vi "CreateTableDB.vi"(8 "error in (no error)":errorcluster) -> (0 "error out":errorcluster)   [LabVIEW 2020, in "Settings.lvlib"]
uses:
  Settings.lvlib
  <vilib>/drjdpowell/SQLite Library/SQL Connection/Open (path).vi
  <vilib>/drjdpowell/SQLite Library/SQL Connection/Open (string).vi
  <vilib>/AdvancedString/Path To Command Line String.vi
  <vilib>/drjdpowell/SQLite Library/SQL Connection/Execute SQL (No results).vi
  <vilib>/drjdpowell/SQLite Library/SQL Connection/Connection.lvclass
  <vilib>/drjdpowell/SQLite Library/SQLite.lvlib
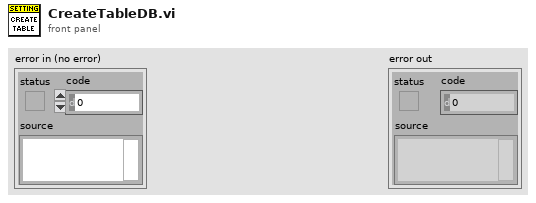
[diagram p1: front panel]
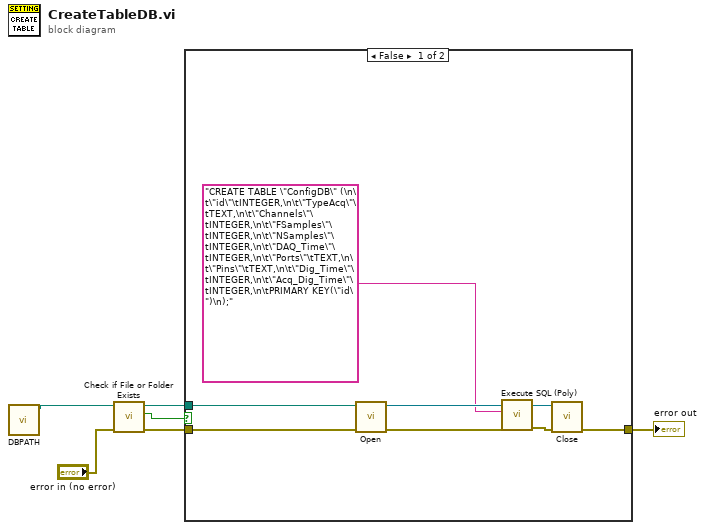
[diagram p0: block diagram]
diagram:
  n1 = call "DBPATH.vi"() -> ("appended path"=w1:path)  [unwired: 11 in]
  n2 = call <vilib>:"Check if File or Folder Exists.vi"("error in (no error)"="error in (no error)", "path"=w1) -> ("error out"=w2:errorcluster, "file or folder exists?"=w4:bool, "dup path"=w5:path)  [unwired: 7 in]
  n3 = case shown="False" w4 {
    tunnel: [w10 w15] -> w6
    tunnel: w5 -> [w7 _]
    tunnel: w2 -> [w8 w15]
    frame False {
      n4 = call-poly <vilib>:"Open.vi"("error in (no error)"=w8, "db file"=w7) -> ("error out"=w14:errorcluster, "SQLite Connection"=w13:refnum<class "Connection.lvclass">)  [unwired: 8 in]
      n5 = call-poly <vilib>:"Execute SQL (Poly).vi"("error in (no error)"=w14, "SQL"="CREATE TABLE \"ConfigDB\" (\n\t\"id\"\tINTEGER,\n\t\"TypeAcq\"\tTEXT,\n\t\"Channels\"\tINTEGER,\n\t\"FSamples\"\tINTEGER,\n\t\"NSamples\"\tINTEGER,\n\t\"DAQ_Time\"\tINTEGER,\n\t\"Ports\"\tTEXT,\n\t\"Pins\"\tTEXT,\n\t\"Dig_Time\"\tINTEGER,\n\t\"Acq_Dig_Time\"\tINTEGER,\n\tPRIMARY KEY(\"id\")\n);", "SQLite Connection in"=w13) -> ("error out"=w12:errorcluster, "SQLite Connection"=w11:refnum<class "Connection.lvclass">)  [unwired: 7 in]
      n6 = call-dynamic "Close.vi"("error in (no error)"=w12, "SQLite Connection in"=w11) -> ("error out"=w10:errorcluster)  [unwired: 9 in]
    }
    frame True {
    }
  }
  "error out" <- w6
